vi "Read Default channels.vi"(8 "error in (no error)":errorcluster, 11 "MagLabGraph in":refnum<class "XY Plot.lvclass">) -> (0 "error out":errorcluster, 2 "Default channels":string[][](array[string]), 3 "MagLabGraph out":refnum<class "XY Plot.lvclass">)   [LabVIEW 2016, in "XY Plot.lvclass"]
uses:
  XY Plot.lvclass
  XY Plot.lvclass/XY Plot.ctl
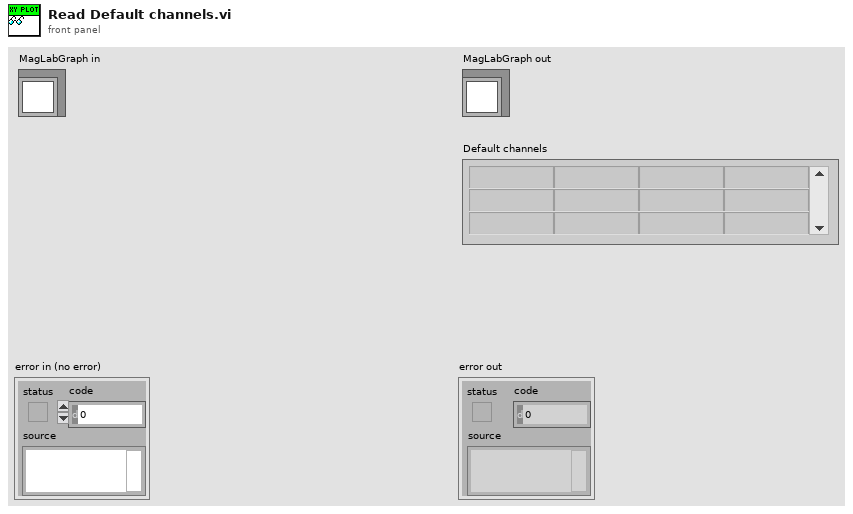
[diagram p1: front panel]
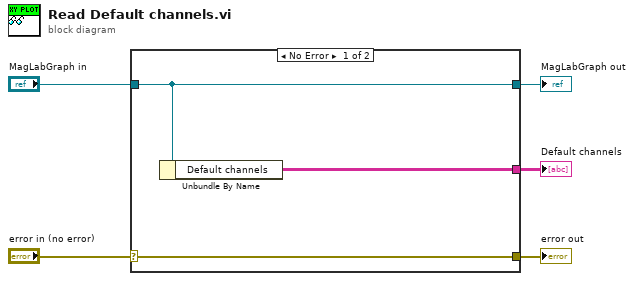
[diagram p0: block diagram]
diagram:
  n1 = case shown="No Error" "error in (no error)" {
    selector: "error in (no error)" -> [w8 w9]
    tunnel: [w8 w9] -> w4
    tunnel: [w7 w10] -> w2
    tunnel: "MagLabGraph in" -> [w7 w10]
    tunnel: [w6 _] -> w1
    frame No Error {
      n2 = Unbundle By Name(w7) -> ("Default channels"=w6:string[][])
    }
    frame Error {
    }
  }
  "error out" <- w4
  "MagLabGraph out" <- w2
  "Default channels" <- w1
